vi "NIPKG List to SBOM Components.vi"(8 "error in (no error)":errorcluster, 11 "nipkg packages":T1[](array[typedef])) -> (0 "error out":errorcluster, 3 "SBOM Components out":refnum<class "CycloneDX Component.lvclass">[](array[class]))   [LabVIEW 2017, in "NIPKG SBOM Support.lvlib"]
doc: "Converts an array of NIPKG information to an array of CycloneDX SBOM components."
uses:
  NIPKG SBOM Support.lvlib
  <vilib>/National Instruments/NIPM API (Beta)/_support/package attributes.ctl
  CycloneDX/CycloneDX Component/CycloneDX Component.lvclass
  <vilib>/National Instruments/NIPM API (Beta)/NIPM_API.lvlib
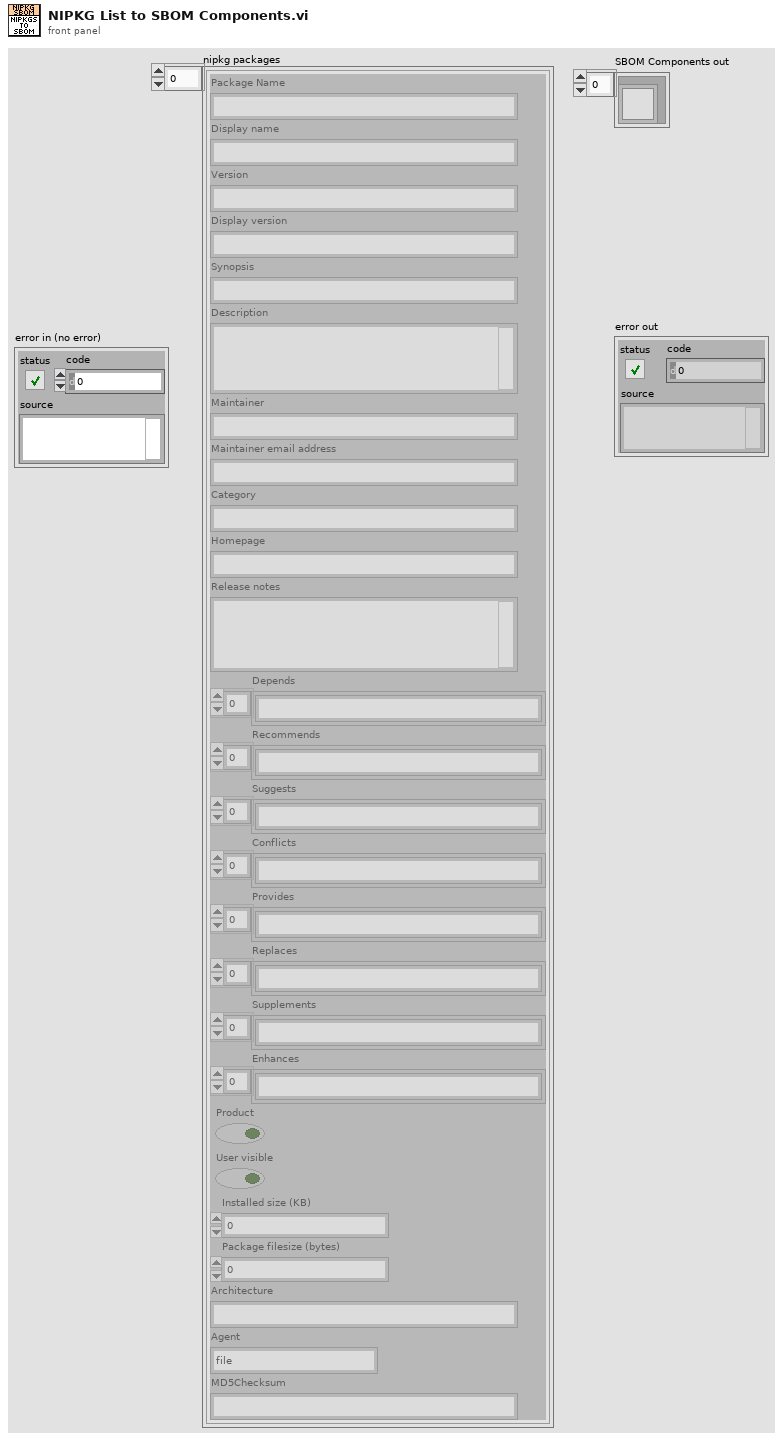
[diagram p1: front panel]
types:
  T1 = typedef "NIPM_API.lvlib/package attributes.ctl" = cluster{"Package Name":string, "Display name":string, "Version":string, "Display version":string, "Synopsis":string, "Description":string, "Maintainer":string, "Maintainer email address":string, "Category":string, "Homepage":string, "Release notes":string, "Depends":string[], "Recommends":string[], "Suggests":string[], "Conflicts":string[], "Provides":string[], "Replaces":string[], "Supplements":string[], "Enhances":string[], "Product":bool, "User visible":bool, "Installed size (KB)":u64, "Package filesize (bytes)":u64, "Architecture":string, "Agent":string, "MD5Checksum":string}
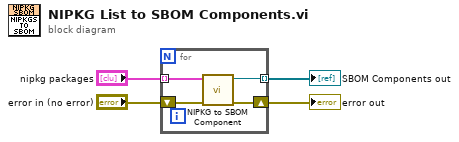
[diagram p0: block diagram]
diagram:
  n1 = for {
    shift-right: [w7] -> w3
    shift-left: "error in (no error)" -> [w8]
    tunnel: [w6] -> w2 mode=indexing
    tunnel: "nipkg packages" -> [w5] mode=indexing
    n2 = call "NIPKG to SBOM Component.vi"("error in (no error)"=w8, "nipkg package attributes"=w5) -> ("error out"=w7:errorcluster, "Component out"=w6:refnum<class "CycloneDX Component.lvclass">)  [unwired: 8 in]
  }
  "SBOM Components out" <- w2
  "error out" <- w3
